vi "lvString to lpString.vi"(11 "LVString":string) -> (3 "LPTSTR String":string)   [LabVIEW 2022 SP3, in "BonTechDetector.lvlib"]
uses:
  BonTechDetector.lvlib
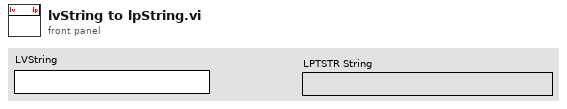
[diagram p1: front panel]
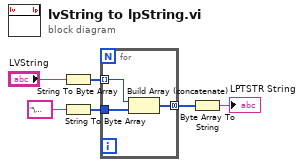
[diagram p0: block diagram]
diagram:
  n1 = String To Byte Array(string="LVString") -> (unsigned byte array=w5:u8[])
  n2 = String To Byte Array(string="\u0000") -> (unsigned byte array=w4:u8[])
  n3 = for {
    tunnel: w5 -> [w9] mode=indexing
    tunnel: w4 -> [w8]
    tunnel: [w7] -> w3 mode=concatenating
    n4 = Build Array (concatenate)(w9, w8) -> (w7:u8[])
  }
  n5 = Byte Array To String(unsigned byte array=w3) -> (string=→"LPTSTR String":string)
